vi "prueba.vi"() -> ()   [LabVIEW 2011]
panel:
  in  "stop":bool
  in  "?":bool
  out "Paro cardiaco":bool
  out "Alarma":bool
  out "Medidor de Corazon":i32(knob) scale=0.0..10.0
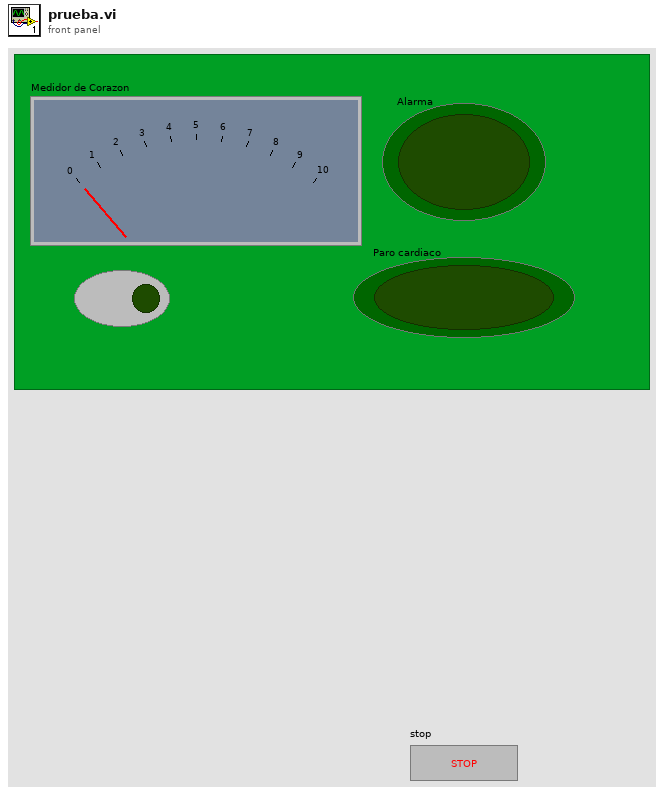
[diagram p1: front panel]
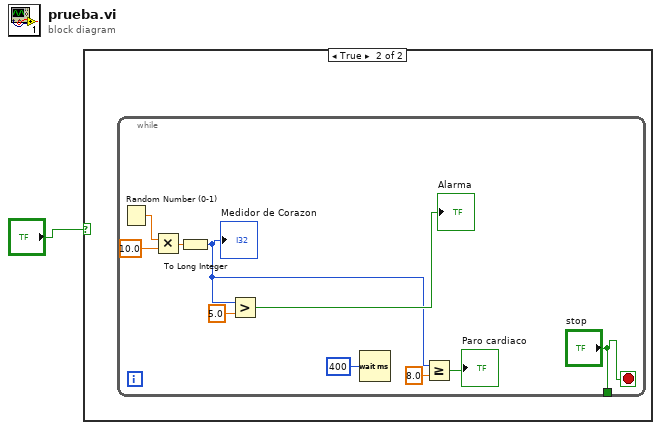
[diagram p0: block diagram]
diagram:
  n1 = case shown="True" "?" {
    frame False {
    }
    frame True {
      n2 = while {
        tunnel: ["stop"] -> _
        stop <- "stop" stop-if-true
        n3 = Random Number (0-1)() -> (number: 0 to 1=w9:dbl)
        n4 = Multiply(x=w9, y=10.0) -> (x*y=w11:dbl)
        n5 = To Long Integer(number=w11) -> (32bit integer=w4:i32)
        "Medidor de Corazon" <- w4
        n6 = Greater?(x=w4, y=5.0) -> (0:→"Alarma":bool)
        n7 = Wait (ms)(milliseconds to wait=u32 400) -> ()  [unwired: 1 out]
        n8 = Greater Or Equal?(x=w4, y=8.0) -> (x >= y?=→"Paro cardiaco":bool)
      }
    }
  }
